vi "qTNS.vi"(0 "System no.":i32=1 min=1 max=4 step=1, 2 "Sensor to query":string[](array[string]), 3 "All sensors?":bool, 4 "Sensor identifier?":bool=TRUE, 5 "error in":errorcluster) -> (14 "Nom. sensor value":dbl[](array[numeric]) format="%.6f", 19 "error out":errorcluster)   [LabVIEW 2026]
doc: "Returns normalized sensor value for the specified sensor number.\n\nC-413 : If All sensors? = TRUE, then Sensor identifier? must be FALSE. Sensors to query comprises all ADC channels of the device: can be a \"genuine\" sensor (sensor integrated in the mechanics) or a \"general purpose\" analog input.\n\nE-709: If All sensors? = TRUE, then Sensor identifier? must be FALSE. Sensors to query comprises all ADC channels of the device: can be the \"genuine\" sensor (sensor integrated in the mechanics, identifier = 1) and the \"general purpose\" analog input (identifier = 2).\n\nE-710: If All sensors? = TRUE, then Sensor identifier? must be TRUE. Command is available in command level 1 only (see CCL.vi and CCL?.vi)\n\nE-712: If All sensors? = TRUE, then Sensor identifier? must be FALSE. Sensors to query comprises all ADC channels of the device: can be a \"genuine\" sensor (sensor integrated in the mechanics) or a \"general purpose\" analog input.\n\nE-725, E-727: If All sensors? = TRUE, then Sensor identifier? must be FALSE. Sensors to query comprises all ADC channels of the device: can be a \"genuine\" sensor (sensor integrated in the mechanics) or a \"general purpose\" analog input.\n\nE-753: If All sensors? = TRUE, then Sensor identifier? must be FALSE. Sensors to query comprises all ADC channels of the device: can be the \"genuine\" sensor (capacitive sensor integrated in the mechanics, identifier = 1) and the \"general purpose\" analog input (identifier = 2).\n\nE-754: If All sensors? = TRUE, then Sensor identifier? must be FALSE. Sensors to query comprises all ADC channels of the device: can be the \"genuine\" sensor (capacitive sensor integrated in the mechanics, identifier = 1, or incremental sensor, identifier = 3) and the \"general purpose\" analog input (identifier = 2).\n\nE-755: If All sensors? = TRUE, then Sensor identifier? must be FALSE. Command not available for E-755.101.\n\nE-761: If All sensors? = TRUE, then Sensor identifier? can be FALSE."
panel:
  # "Returns normalized sensor value for the specified sensor number."
  # "If all sensors: use"
  # "Query"
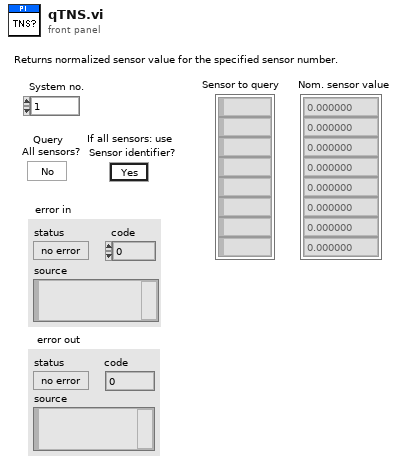
[diagram p1: front panel]
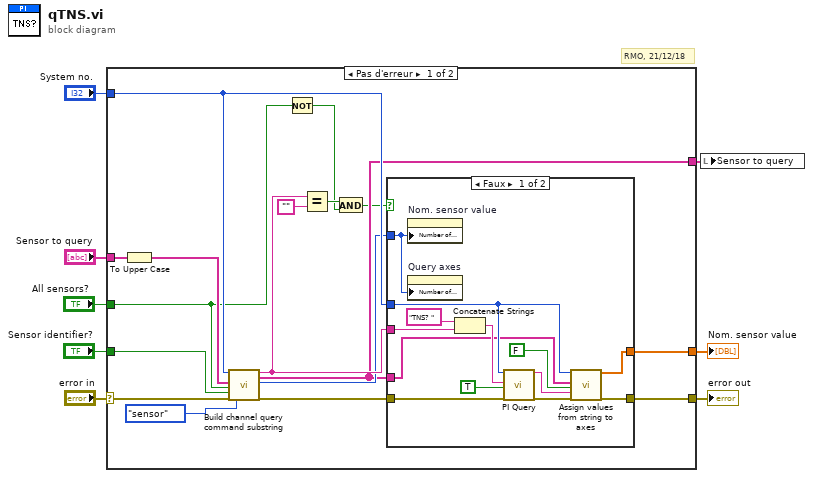
[diagram p0: block diagram]
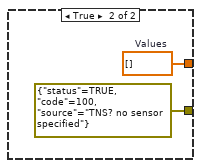
[diagram p2: hidden frame]
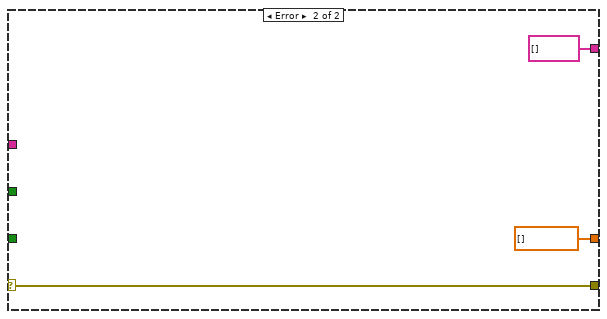
[diagram p3: hidden frame]
diagram:
  # "RMO, 21/12/18"
  n1 = case shown="Pas d'erreur" "error in" {
    selector: "error in" -> [w11 w41]
    tunnel: [w25 dbl[] [] ("Values")] -> w8
    tunnel: "Sensor to query" -> [w24 _]
    tunnel: [w10 w41] -> w6
    tunnel: "Sensor identifier?" -> [w15 _]
    tunnel: "System no." -> [w18 _]
    tunnel: [w12 string[] [] ("Axes to query out")] -> w3
    tunnel: "All sensors?" -> [w16 _]
    frame No Error {
      n2 = To Upper Case(1:w24) -> (0:w17:string[])
      n3 = call "Build channel query command substring.vi"("System no."=w18, "Channels to query in"=w17, "Query\nAll channels?"=w16, "For all channels: use\nChannel identifier?"=w15, "error in"=w11, "Channel type"=enum16{"piezo", "sensor"}."sensor") -> ("Command substring"=w14:string, "Channels to query out"=w12:string[], "Number of rows"=w13:u32, "error out"=w19:errorcluster)  [unwired: 1 in, 9 out]
      n4 = Not(x=w16) -> (.not. x?=w21:bool)
      n5 = Equal?(x=w14, y="" ("x")) -> (x = y?=w22:bool)
      n6 = And(x=w22, y=w21) -> (x .and. y?=w9:bool)
      n7 = case shown="Faux" w9 {
        tunnel: [w35 w39] -> w25
        tunnel: w19 -> [w34 _]
        tunnel: w18 -> [w33 _]
        tunnel: w14 -> [w32 _]
        tunnel: w13 -> [w31 _]
        tunnel: w12 -> [w30 _]
        tunnel: [w28 errorcluster {"status"=TRUE, "code"=100, "source"="TNS? no sensor specified"} ("error out")] -> w10
        frame False {
          n8 = property on="Nom. sensor value" class="Tabl (strict)"("Number of Rows"=w31) -> ()  [unwired: 2 in, 2 out]
          n9 = property on="Query axes" class="Tabl (strict)"("Number of Rows"=w31) -> ()  [unwired: 2 in, 2 out]
          n10 = Concatenate Strings("TNS? ", w32) -> (w36:string)
          n11 = call "PI Query.vi"("System no."=w33, "String to send"=w36, "Attach termination char.?"=TRUE ("Attach Linefeed?"), "error in"=w34) -> ("String read"=w26:string, "error out"=w27:errorcluster)  [unwired: 3 in, 11 out]
          n12 = call "Assign values from string to axes.vi"("System no."=w33, "Queried axes"=w30, "All axes queried?"=FALSE, "Input String"=w26, "error in"=w27) -> ("Values"=w35:dbl[], "error out"=w28:errorcluster)  [unwired: 4 in, 9 out]
        }
        frame True {
          w39 = dbl[] []  # Values
        }
      }
    }
    frame Error {
    }
  }
  "error out" <- w6
  "Nom. sensor value" <- w8
  n13 = local write "Sensor to query"(w3) -> ()
